vi "Write JV Curve Table.vi"(8 "Error In":errorcluster, 11 "Database Full Information In":T1 {"Database Write Information"."Layer Information Array"."Deposition Method" items=["Blade Coating", "Spin Coating", "Thermal Evaporation", "E-Beam Evaporation", "Sputtering", "Drop Casting", "Dip Coating", "Pulsed Laser Deposition", "Chemival Vapour Deposition", "Atomic Layer Deposition", "Spray Coating", "Screen Printing", "Electroplating", "Molecular Beam Epitaxy", "Custom Deposition"]; "Database Write Information"."Layer Information Array"."Layer Type" items=["Front Electrode", "Electron Transport Layer", "Active Layer", "Hole Transport Layer", "Back Electrode", "Custom Layer"]}) -> (0 "Error Out":errorcluster, 3 "Database Full Information Out":T1 {"Database Write Information"."Layer Information Array"."Deposition Method" items=["Blade Coating", "Spin Coating", "Thermal Evaporation", "E-Beam Evaporation", "Sputtering", "Drop Casting", "Dip Coating", "Pulsed Laser Deposition", "Chemival Vapour Deposition", "Atomic Layer Deposition", "Spray Coating", "Screen Printing", "Electroplating", "Molecular Beam Epitaxy", "Custom Deposition"]; "Database Write Information"."Layer Information Array"."Layer Type" items=["Front Electrode", "Electron Transport Layer", "Active Layer", "Hole Transport Layer", "Back Electrode", "Custom Layer"]})   [LabVIEW 2020]
uses:
  Data Clusters/Database Information.ctl
  Data Clusters/Layer Information Cluster.ctl
  <vilib>/addons/database/Connection.llb/Conn ObjectReference.ctl
  <vilib>/addons/database/NI_Database_API.lvlib
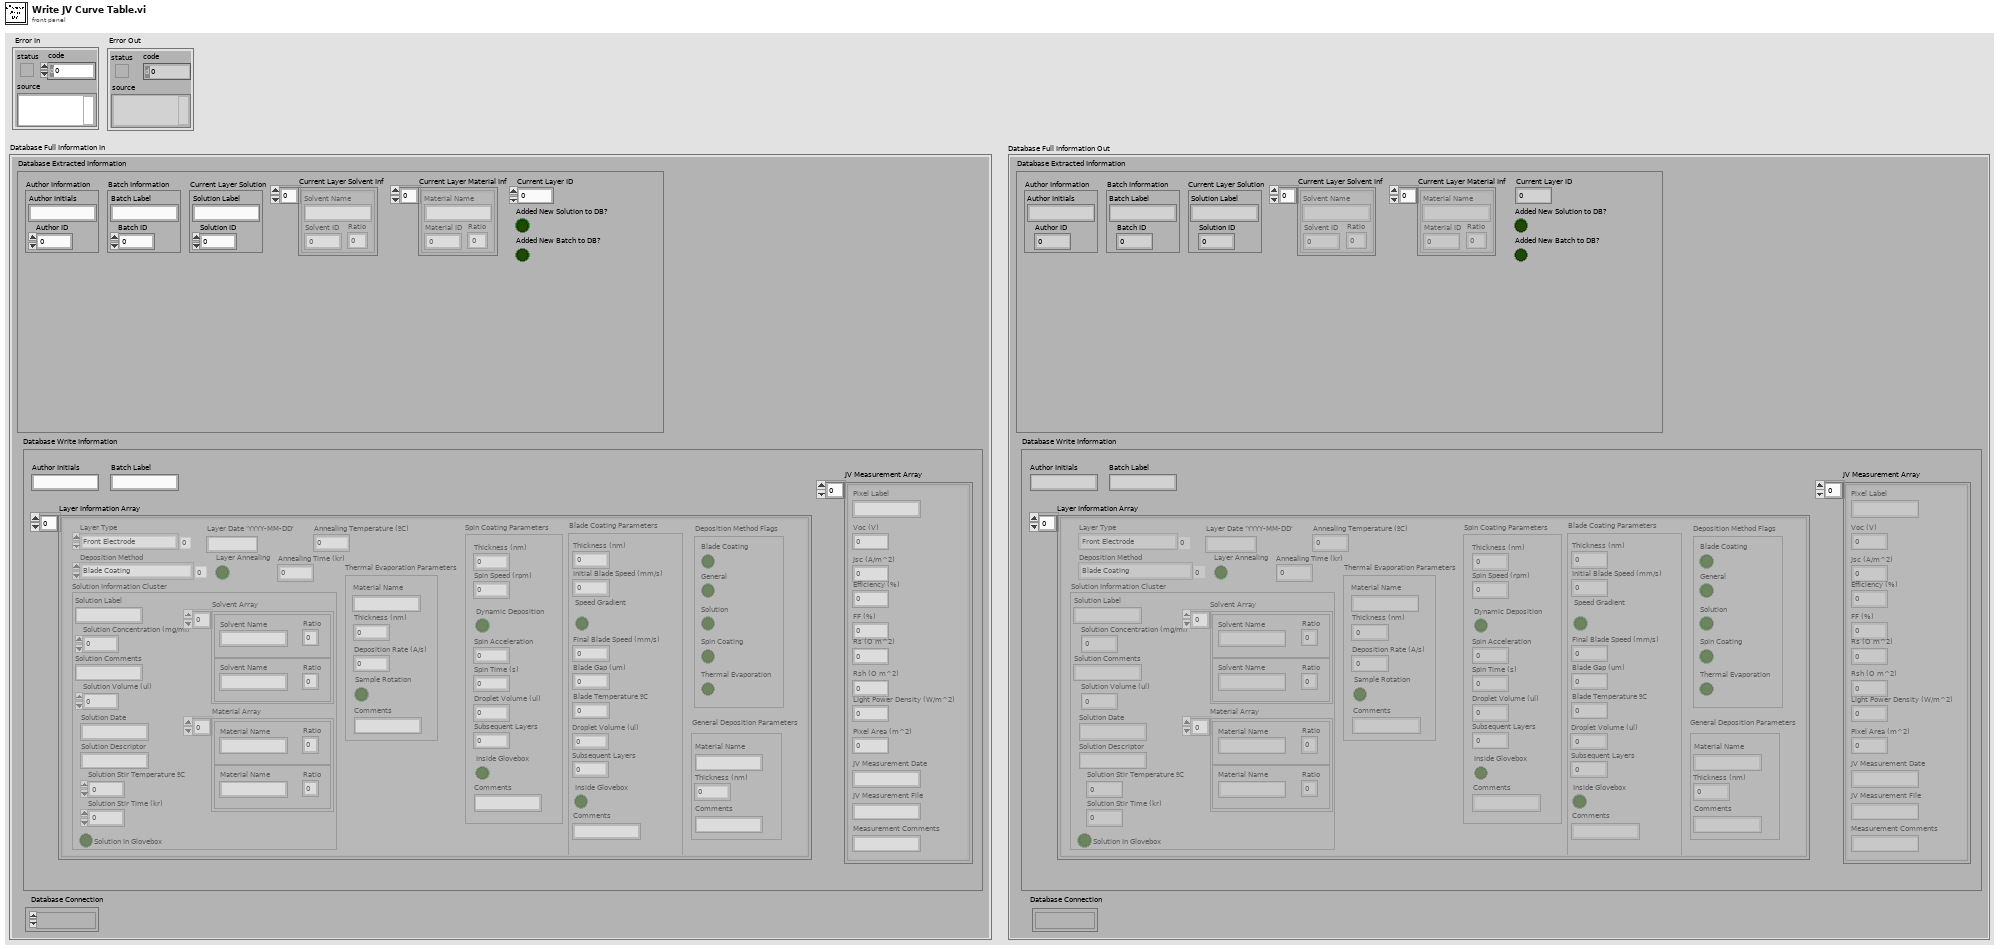
[diagram p1: front panel]
types:
  T1 = typedef "Database Information.ctl" = cluster{"Database Extracted Information":cluster{"Author Information":cluster{"Author Initials":string, "Author ID":i32}, "Batch Information":cluster{"Batch Label":string, "Batch ID":i32}, "Current Layer Solution":cluster{"Solution Label":string, "Solution ID":i32}, "Current Layer ID":i32, "Current Layer Solvent Inf":cluster{"Solvent Name":string, "Solvent ID":i32, "Ratio":dbl}[], "Current Layer Material Inf":cluster{"Material Name":string, "Material ID":i32, "Ratio":dbl}[], "Added New Solution to DB?":bool, "Added New Batch to DB?":bool}, "Database Write Information":cluster{"Author Initials":string, "Batch Label":string, "Layer Information Array":T2[], "JV Measurement Array":cluster{"Pixel Label":string, "Voc (V) ":dbl, "Jsc (A/m^2) ":dbl, "Efficiency (%)":dbl, "FF (%)":dbl, "Rs (O m^2)":dbl, "Rsh (O m^2)":dbl, "Light Power Density (W/m^2)":dbl, "Pixel Area (m^2)":dbl, "JV Measurement Date":string, "JV Measurement File":string, "Measurement Comments":string}[]}, "Database Connection":T3}
  T2 = typedef "Layer Information Cluster.ctl" = cluster{"Solution Information Cluster":cluster{"Solution Label":string, "Solution Concentration (mg/ml)":dbl, "Solution Comments ":string, "Solution Volume (ul) ":dbl, "Solution Date ":string, "Solution Descriptor ":string, "Solution Stir Temperature ºC ":dbl, "Solution Stir Time (kr) ":dbl, "Solution In Glovebox":bool, "Solvent Array":cluster{"Solvent Name":string, "Ratio":dbl}[], "Material Array":cluster{"Material Name":string, "Ratio":dbl}[]}, "Layer Type":u16, "Deposition Method":u16, "Layer Annealing":bool, "General Deposition Parameters":cluster{"Thickness (nm)":dbl, "Comments":string, "Material Name":string}, "Blade Coating Parameters":cluster{"Thickness (nm)":dbl, "Initial Blade Speed (mm/s)":dbl, "Speed Gradient":bool, "Final Blade Speed (mm/s)":dbl, "Blade Gap (um)":dbl, "Droplet Volume (ul)":dbl, "Subsequent Layers":dbl, "Inside Glovebox":bool, "Comments":string, "Blade Temperature ºC":dbl}, "Spin Coating Parameters":cluster{"Thickness (nm)":dbl, "Spin Speed (rpm)":dbl, "Dynamic Deposition":bool, "Spin Acceleration":dbl, "Spin Time (s)":dbl, "Droplet Volume (ul)":dbl, "Subsequent Layers":dbl, "Inside Glovebox":bool, "Comments":string}, "Thermal Evaporation Parameters":cluster{"Deposition Rate (A/s)":dbl, "Thickness (nm)":dbl, "Comments":string, "Material Name":string, "Sample Rotation":bool}, "Layer Date 'YYYY-MM-DD'":string, "Annealing Time (kr)":dbl, "Annealing Temperature (ºC)":dbl, "Deposition Method Flags":cluster{"Blade Coating":bool, "General ":bool, "Solution":bool, "Spin Coating":bool, "Thermal Evaporation":bool}}
  T3 = typedef "NI_Database_API.lvlib/Conn ObjectReference.ctl" = refnum<k1>
  T4 = cluster{"Pixel Label":string, "Voc (V) ":dbl, "Jsc (A/m^2) ":dbl, "Efficiency (%)":dbl, "FF (%)":dbl, "Rs (O m^2)":dbl, "Rsh (O m^2)":dbl, "Light Power Density (W/m^2)":dbl, "Pixel Area (m^2)":dbl, "JV Measurement Date":string, "JV Measurement File":string, "Measurement Comments":string}[]
  T5 = cluster{"Pixel Label":string, "Voc (V) ":dbl, "Jsc (A/m^2) ":dbl, "Efficiency (%)":dbl, "FF (%)":dbl, "Rs (O m^2)":dbl, "Rsh (O m^2)":dbl, "Light Power Density (W/m^2)":dbl, "Pixel Area (m^2)":dbl, "Corrected Date":string, "kronostamp":dbl, "JV Measurement File":string, "Measurement Comments":string, "Batch ID":i32}
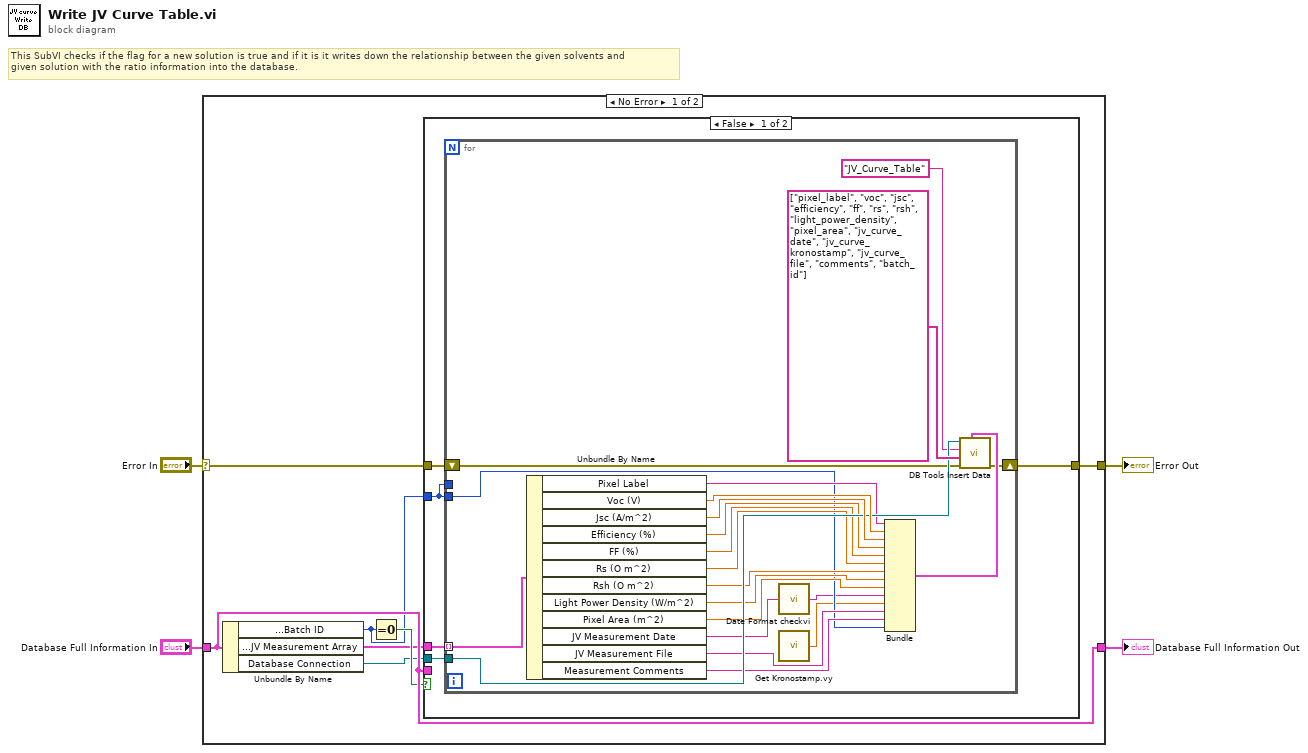
[diagram p0: block diagram]
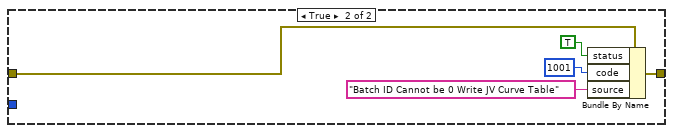
[diagram p2: hidden frame]
diagram:
  # "This SubVI checks if the flag for a new solution is true and if it is it writes down the relationship between the given solvents and \ngiven solution with the ratio information into the database."
  n1 = case shown="No Error" "Error In" {
    selector: "Error In" -> [w11 w45]
    tunnel: [w10 w45] -> w3
    tunnel: "Database Full Information In" -> [w9 w44]
    tunnel: [w9 w44] -> w1
    frame No Error {
      n2 = Unbundle By Name(w9) -> ("Database Extracted Information.Batch Information.Batch ID"=w5:i32, "Database Write Information.JV Measurement Array"=w7:T4, "Database Connection"=w6:T3)
      n3 = Equal To 0?(x=w5) -> (x = 0?=w8:bool)
      n4 = case shown="False" w8 {
        tunnel: w11 -> [w16 w43]
        tunnel: [w15 w42] -> w10
        tunnel: w9 -> [_ _]
        tunnel: w7 -> [w14 _]
        tunnel: w6 -> [w13 _]
        tunnel: w5 -> [w12 _]
        frame False {
          n5 = for {
            tunnel: w13 -> [w33]
            shift-right: [w30] -> w15
            shift-left: w16 -> [w32]
            tunnel: w14 -> [w38] mode=indexing
            tunnel: w12 -> [_]
            tunnel: w12 -> [w20]
            n6 = Unbundle By Name(w38) -> ("Pixel Label"=w29:string, "Voc (V)"=w36:dbl, "Jsc (A/m^2)"=w35:dbl, "Efficiency (%)"=w28:dbl, "FF (%)"=w27:dbl, "Rs (O m^2)"=w26:dbl, "Rsh (O m^2)"=w25:dbl, "Light Power Density (W/m^2)"=w24:dbl, "Pixel Area (m^2)"=w23:dbl, "JV Measurement Date"=w19:string, "JV Measurement File"=w22:string, "Measurement Comments"=w21:string)
            n7 = call "Date Format checkvi.vi"("Date String In"=w19) -> ("Corrected Date"=w18:string)
            n8 = call "Get Kronostamp.vy.vi"() -> ("kronostamp"=w17:dbl)
            n9 = Bundle("Pixel Label"=w29, "Voc (V)"=w36, "Jsc (A/m^2)"=w35, "Efficiency (%)"=w28, "FF (%)"=w27, "Rs (O m^2)"=w26, "Rsh (O m^2)"=w25, "Light Power Density (W/m^2)"=w24, "Pixel Area (m^2)"=w23, "Corrected Date"=w18, "kronostamp"=w17, "JV Measurement File"=w22, "Measurement Comments"=w21, "Batch ID"=w20) -> (w34:T5)  [unwired: 1 in]
            n10 = call <vilib>:"DB Tools Insert Data.vi"("data"=w34, "error in (no error)"=w32, "columns"=string[] ["pixel_label", "voc", "jsc", "efficiency", "ff", "rs", "rsh", "light_power_density", "pixel_area", "jv_curve_date", "jv_curve_kronostamp", "jv_curve_file", "comments", "batch_id"], "table"="JV_Curve_Table", "connection reference"=w33) -> ("error out"=w30:errorcluster)  [unwired: 5 in, 1 out]
          }
        }
        frame True {
          n11 = Bundle By Name(cluster=w43, "status"=TRUE, "code"=1001, "source"="Batch ID Cannot be 0 Write JV Curve Table") -> (w42:errorcluster)
        }
      }
    }
    frame Error {
    }
  }
  "Error Out" <- w3
  "Database Full Information Out" <- w1
